vi "WT 2X0 Harmonic 6 Item Measurements.vi"(8 "error in (no error)":errorcluster, 11 "VISA resource name":refnum<visa-resource-name>) -> (0 "error out":errorcluster, 1 "appended array":string[][](array[string]), 2 "Output Array":sgl[](array[numeric]), 3 "VISA resource name out":refnum<visa-resource-name>)   [LabVIEW 2010]
doc: "This VI measures Voltage, THD, Power Factor, Frequency, Current, and Power. This VI outputs the information in a string array with labels.\n\nIMPORTANT!!!: Harmonics configuration must be set up and enabled prior to calling this VI"
uses:
  instr.lib/Yokogawa WT200 Series/Yokogawa WT200 Series.lvlib
panel:
  out "Power":sgl
  out "Current":sgl
  out "Frequency":sgl
  out "Power Factor":sgl
  out "THD":sgl
  out "Voltage":sgl
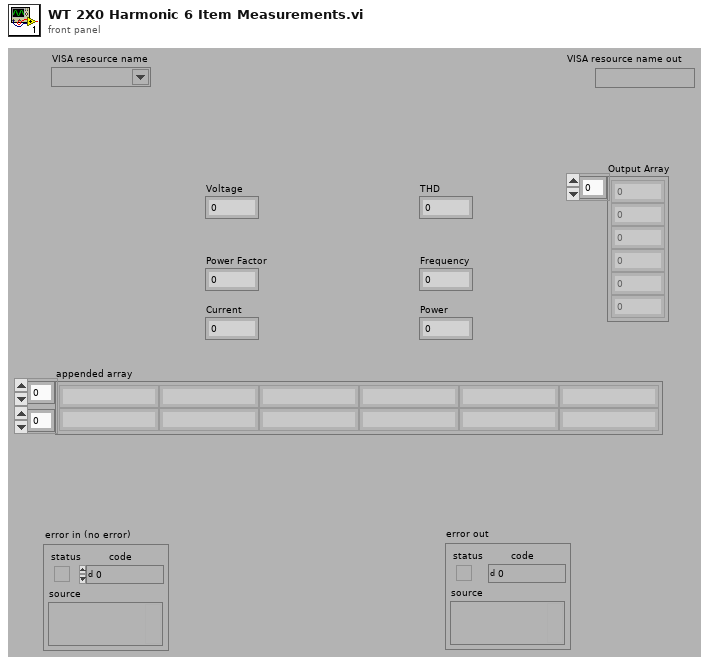
[diagram p1: front panel]
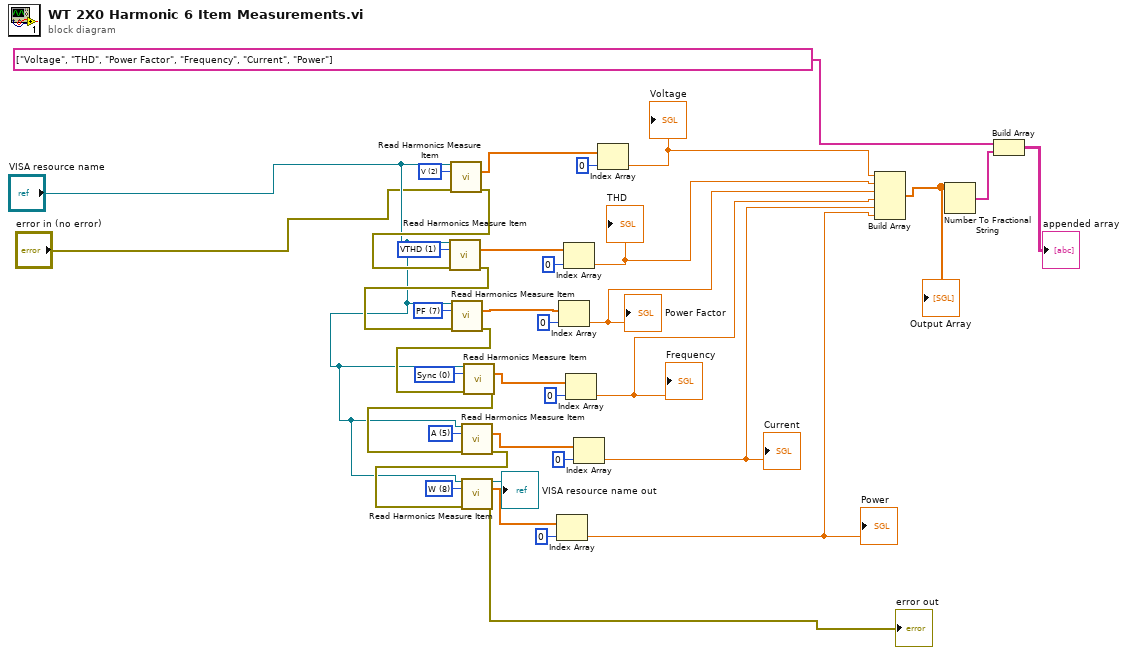
[diagram p0: block diagram]
diagram:
  w22 = u16 8 items=["Sync", "VTHD", "V", "VCON", "ATHD", "A", "ACON", "PF", "W", "WCON", "Vdeg", "Adeg"] ("Harmonics Item (2: V)")
  w23 = u16 5 items=["Sync", "VTHD", "V", "VCON", "ATHD", "A", "ACON", "PF", "W", "WCON", "Vdeg", "Adeg"] ("Harmonics Item (2: V)")
  w31 = u16 0 items=["Sync", "VTHD", "V", "VCON", "ATHD", "A", "ACON", "PF", "W", "WCON", "Vdeg", "Adeg"] ("Harmonics Item (2: V)")
  w32 = u16 7 items=["Sync", "VTHD", "V", "VCON", "ATHD", "A", "ACON", "PF", "W", "WCON", "Vdeg", "Adeg"] ("Harmonics Item (2: V)")
  w33 = u16 1 items=["Sync", "VTHD", "V", "VCON", "ATHD", "A", "ACON", "PF", "W", "WCON", "Vdeg", "Adeg"] ("Harmonics Item (2: V)")
  w34 = u16 2 items=["Sync", "VTHD", "V", "VCON", "ATHD", "A", "ACON", "PF", "W", "WCON", "Vdeg", "Adeg"] ("Harmonics Item (2: V)")
  n1 = call "Read Harmonics Measure Item.vi"("VISA resource name"="VISA resource name", "Harmonics Item (2: V)"=w34, "error in (no error)"="error in (no error)") -> ("Data"=w24:sgl[], "error out"=w37:errorcluster)  [unwired: 10 in, 1 out]
  n2 = call "Read Harmonics Measure Item.vi"("VISA resource name"="VISA resource name", "Harmonics Item (2: V)"=w33, "error in (no error)"=w37) -> ("Data"=w21:sgl[], "error out"=w36:errorcluster)  [unwired: 10 in, 1 out]
  n3 = call "Read Harmonics Measure Item.vi"("VISA resource name"="VISA resource name", "Harmonics Item (2: V)"=w32, "error in (no error)"=w36) -> ("Data"=w20:sgl[], "error out"=w35:errorcluster)  [unwired: 10 in, 1 out]
  n4 = call "Read Harmonics Measure Item.vi"("VISA resource name"="VISA resource name", "Harmonics Item (2: V)"=w31, "error in (no error)"=w35) -> ("Data"=w19:sgl[], "error out"=w17:errorcluster)  [unwired: 10 in, 1 out]
  n5 = call "Read Harmonics Measure Item.vi"("VISA resource name"="VISA resource name", "Harmonics Item (2: V)"=w23, "error in (no error)"=w17) -> ("Data"=w14:sgl[], "error out"=w16:errorcluster)  [unwired: 10 in, 1 out]
  n6 = call "Read Harmonics Measure Item.vi"("VISA resource name"="VISA resource name", "Harmonics Item (2: V)"=w22, "error in (no error)"=w16) -> ("VISA resource name out"=→"VISA resource name out":refnum<visa-resource-name>, "Data"=w18:sgl[], "error out"=→"error out":errorcluster)  [unwired: 10 in]
  n7 = Index Array(array=w18, index=0) -> (element=w8:sgl)
  "Power" <- w8
  n8 = Index Array(array=w20, index=0) -> (element=w11:sgl)
  "Power Factor" <- w11
  n9 = Index Array(array=w21, index=0) -> (element=w12:sgl)
  "THD" <- w12
  n10 = Index Array(array=w19, index=0) -> (element=w10:sgl)
  "Frequency" <- w10
  n11 = Index Array(array=w14, index=0) -> (element=w9:sgl)
  "Current" <- w9
  n12 = Index Array(array=w24, index=0) -> (element=w13:sgl)
  "Voltage" <- w13
  n13 = Build Array(w13, w12, w11, w10, w9, w8) -> (w7:sgl[])
  "Output Array" <- w7
  n14 = Number To Fractional String(number=w7) -> (F-format string=w6:string[])  [unwired: 3 in]
  n15 = Build Array(string[] ["Voltage", "THD", "Power Factor", "Frequency", "Current", "Power"], w6) -> (→"appended array":string[][])
